vi "Move piezo.vi"(7 "error in (no error)":errorcluster, 8 "MOVE TO [MICRON]":dbl=1.0 format="%0.2f", 9 "notifier out":refnum<notifier>, 10 "Hardware Configuration":T1) -> (0 "error out":errorcluster, 3 "Hardware Configuration 2":T1)   [LabVIEW 2013, in "Piezo.lvlib"]
uses:
  Piezo/Piezo.lvlib
  Hardware Configuration Piezo.ctl
  Piezo/Piezo display.ctl
  <vilib>/DAQmx/create/channels.llb/DAQmx Create Channel (AO-Voltage-Basic).vi
  <vilib>/DAQmx/write.llb/DAQmx Write (Analog DBL 1Chan 1Samp).vi
panel:
  out "PiezoPosition":sgl
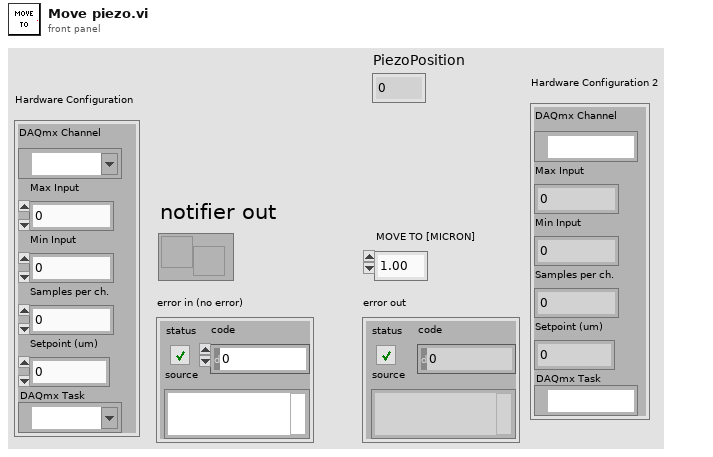
[diagram p1: front panel]
types:
  T1 = typedef "Piezo.lvlib/Hardware Configuration Piezo.ctl" = cluster{"DAQmx Channel":tag, "Max Input":dbl, "Min Input":dbl, "Samples per ch.":dbl, "Setpoint (um)":dbl, "DAQmx Task":refnum<k21>}
  T2 = typedef "Piezo.lvlib/Piezo display.ctl" = cluster{"PiezoPosition":sgl, "Counter Time":i32}
  T3 = cluster{"physical channels":tag, "MAX   VOLTAGE":dbl, "MIN   VOLTAGE":dbl}
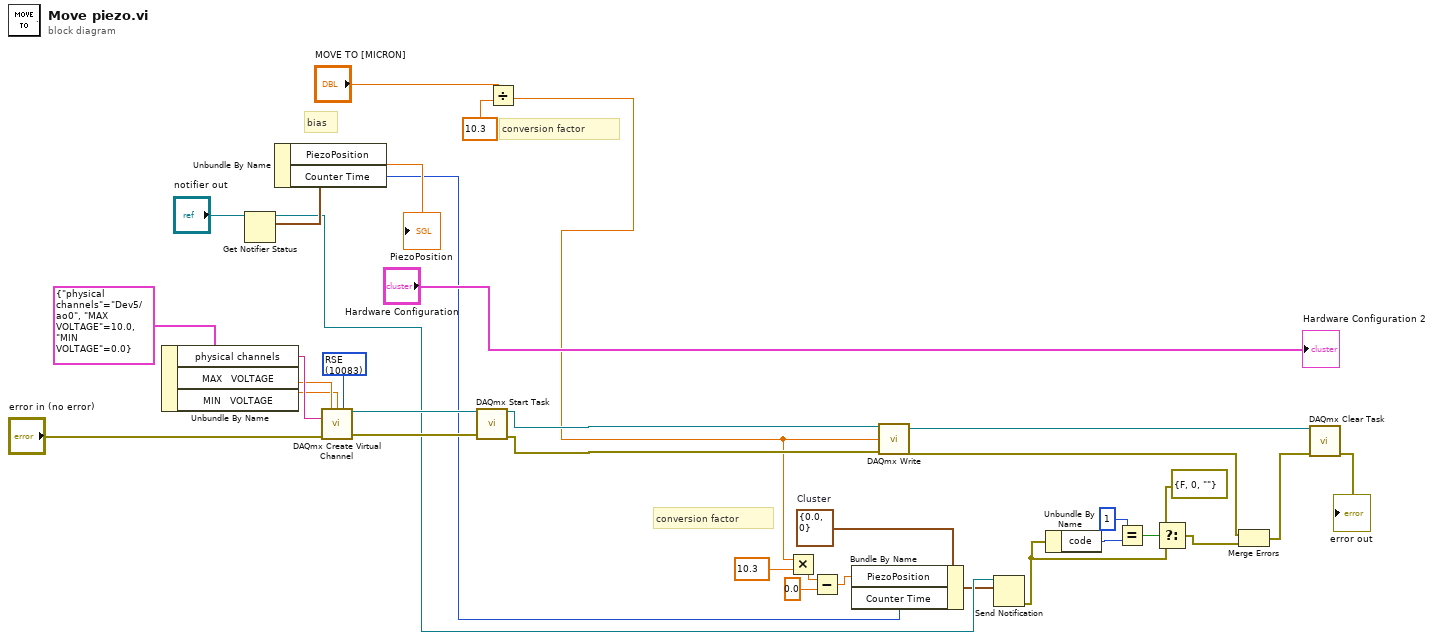
[diagram p0: block diagram]
diagram:
  w13 = T2 {"PiezoPosition"=0.0, "Counter Time"=0}  # Cluster
  w31 = 10083 items=["Default"=-1, "RSE"=10083, "Differential"=10106, "Pseudodifferential"=12529] ("output terminal configuration")
  # "conversion factor"
  # "bias"
  # "conversion factor"
  n1 = Unbundle By Name(T3 {"physical channels"="Dev5/ao0", "MAX   VOLTAGE"=10.0, "MIN   VOLTAGE"=0.0} ("Cluster")) -> ("physical channels"=w27:tag, "MAX   VOLTAGE"=w26:dbl, "MIN   VOLTAGE"=w25:dbl)
  n2 = Get Notifier Status(notifier="notifier out") -> (notifier out=w17:refnum<notifier>, current notification=w33:T2)  [unwired: 1 in, 3 out]
  n3 = Unbundle By Name(w33) -> ("PiezoPosition"=→"PiezoPosition":sgl, "Counter Time"=w16:i32)
  n4 = call-poly <vilib>:"DAQmx Create Virtual Channel.vi"("maximum value"=w26, "minimum value"=w25, "output terminal configuration"=w31, "physical channels"=w27, "error in"="error in (no error)") -> ("task out"=w30:refnum<k21>, "error out"=w29:errorcluster)  [unwired: 9 in]
  n5 = call <vilib>:"DAQmx Start Task.vi"("task/channels in"=w30, "error in"=w29) -> ("task out"=w21:refnum<k21>, "error out"=w20:errorcluster)  [unwired: 12 in]
  n6 = Divide(x="MOVE TO [MICRON]", y=10.3) -> (x/y=w1:dbl)
  n7 = Multiply(x=w1, y=10.3) -> (x*y=w3:dbl)
  n8 = Subtract(x=w3, y=0.0) -> (x-y=w4:dbl)
  n9 = Bundle By Name(cluster=w13, "PiezoPosition"=w4, "Counter Time"=w16) -> (w14:T2)
  n10 = call-poly <vilib>:"DAQmx Write.vi"("task/channels in"=w21, "data"=w1, "error in"=w20) -> ("task out"=w23:refnum<k21>, "error out"=w8:errorcluster)  [unwired: 10 in, 1 out]
  n11 = Send Notification(notification=w14, notifier=w17) -> (error out=w7:errorcluster)  [unwired: 1 in, 1 out]
  n12 = Unbundle By Name(w7) -> ("code"=w12:i32)
  n13 = Equal?(x=1, y=w12) -> (x = y?=w10:bool)
  n14 = Select(t=errorcluster {"status"=FALSE, "code"=0, "source"=""} ("error constant"), s=w10, f=w7) -> (s? t:f=w6:errorcluster)
  n15 = Merge Errors(w8, w6) -> (w22:errorcluster)
  n16 = call <vilib>:"DAQmx Clear Task.vi"("task in"=w23, "error in"=w22) -> ("error out"=→"error out":errorcluster)  [unwired: 13 in]
  "Hardware Configuration 2" <- "Hardware Configuration"
